vi "663xA Set Mask Register.vi"(0 "VISA resource name":refnum<visa-resource-name>, 1 "normal mode (F:off)":bool, 2 "fast mode (F:off)":bool, 3 "-cc mode (F:off)":bool, 4 "remote inhibit (F:off)":bool, 5 "error in (no error)":errorcluster, 6 "error (F:off)":bool, 7 "output unregulated (F:off)":bool, 8 "overcurrent (F:off)":bool, 9 "+cc mode (F:off)":bool, 10 "overtemperature (F:off)":bool, 11 "cv mode (F:off)":bool, 12 "overvoltage (F:off)":bool) -> (14 "VISA resource name out":refnum<visa-resource-name>, 19 "error out":errorcluster)   [LabVIEW 2020, in "Agilent 6XXX Series.lvlib"]
doc: "This function sets the mask register which specifies which bits in the status register are enabled to set bits in the fault register. Basically, this function allows the operator to define which conditions are fault conditions."
uses:
  <instrlib>/Agilent 6XXX Series/Agilent 6XXX Series.lvlib
panel:
  # "HP663XA series only"
  # "Set Mask for.."
  # "on\noff"
  # "on\noff"
  # "on\noff"
  # "on\noff"
  # "on\noff"
  # "on\noff"
  # "on\noff"
  # "on\noff"
  # "on\noff"
  # "on\noff"
  # "on\noff"
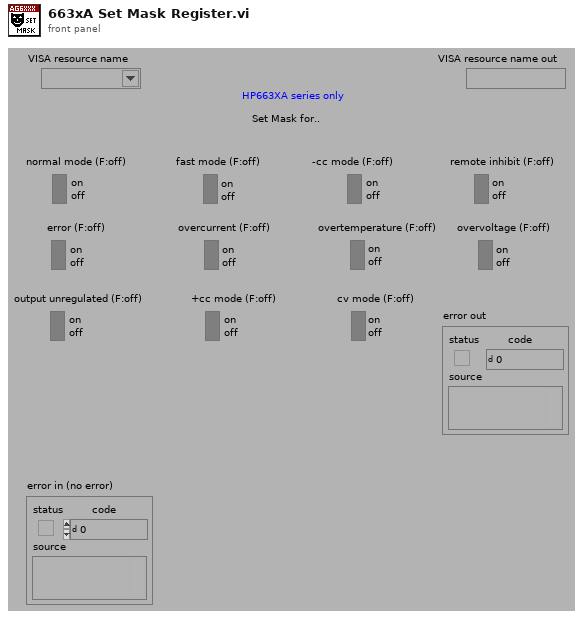
[diagram p1: front panel]
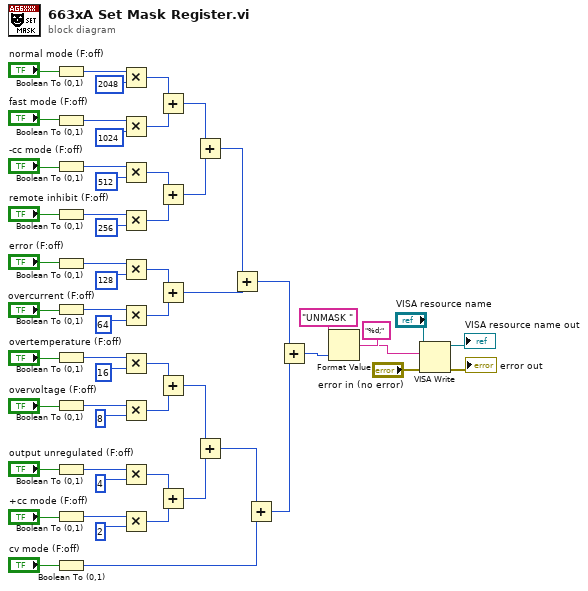
[diagram p0: block diagram]
diagram:
  n1 = Boolean To (0,1)(Boolean="normal mode (F:off)") -> (0, 1=w12:i16)
  n2 = Boolean To (0,1)(Boolean="fast mode (F:off)") -> (0, 1=w13:i16)
  n3 = Boolean To (0,1)(Boolean="-cc mode (F:off)") -> (0, 1=w14:i16)
  n4 = Boolean To (0,1)(Boolean="remote inhibit (F:off)") -> (0, 1=w51:i16)
  n5 = Boolean To (0,1)(Boolean="error (F:off)") -> (0, 1=w50:i16)
  n6 = Boolean To (0,1)(Boolean="overcurrent (F:off)") -> (0, 1=w49:i16)
  n7 = Boolean To (0,1)(Boolean="overtemperature (F:off)") -> (0, 1=w48:i16)
  n8 = Boolean To (0,1)(Boolean="overvoltage (F:off)") -> (0, 1=w47:i16)
  n9 = Boolean To (0,1)(Boolean="output unregulated (F:off)") -> (0, 1=w46:i16)
  n10 = Boolean To (0,1)(Boolean="+cc mode (F:off)") -> (0, 1=w45:i16)
  n11 = Boolean To (0,1)(Boolean="cv mode (F:off)") -> (0, 1=w31:i16)
  n12 = Multiply(x=w12, y=i16 2048) -> (x*y=w18:i16)
  n13 = Multiply(x=w13, y=i16 1024) -> (x*y=w19:i16)
  n14 = Multiply(x=w14, y=i16 512) -> (x*y=w8:i16)
  n15 = Multiply(x=w51, y=i16 256) -> (x*y=w7:i16)
  n16 = Multiply(x=w50, y=i16 128) -> (x*y=w6:i16)
  n17 = Multiply(x=w49, y=i16 64) -> (x*y=w5:i16)
  n18 = Multiply(x=w48, y=i16 16) -> (x*y=w37:i16)
  n19 = Multiply(x=w47, y=i16 8) -> (x*y=w36:i16)
  n20 = Multiply(x=w46, y=i16 4) -> (x*y=w35:i16)
  n21 = Multiply(x=w45, y=i16 2) -> (x*y=w34:i16)
  n22 = Add(x=w18, y=w19) -> (x+y=w20:i16)
  n23 = Add(x=w8, y=w7) -> (x+y=w4:i16)
  n24 = Add(x=w6, y=w5) -> (x+y=w3:i16)
  n25 = Add(x=w37, y=w36) -> (x+y=w32:i16)
  n26 = Add(x=w35, y=w34) -> (x+y=w33:i16)
  n27 = Add(x=w20, y=w4) -> (x+y=w2:i16)
  n28 = Add(x=w32, y=w33) -> (x+y=w30:i16)
  n29 = Add(x=w2, y=w3) -> (x+y=w29:i16)
  n30 = Add(x=w30, y=w31) -> (x+y=w28:i16)
  n31 = Add(x=w29, y=w28) -> (x+y=w27:i16)
  n32 = Format Value(string ("")="UNMASK ", format string="%d;", value (0)=w27) -> (output string=w1:string)
  n33 = VISA Write(VISA resource name="VISA resource name", write buffer=w1, error in (no error)="error in (no error)") -> (VISA resource name out=→"VISA resource name out":refnum<visa-resource-name>, error out=→"error out":errorcluster)  [unwired: 1 out]
